vi "Read Message.vi"(11 "LogMessage In":refnum<class "LogMessage.lvclass">) -> (2 "Message":string, 3 "LogMessage Out":refnum<class "LogMessage.lvclass">)   [LabVIEW 2019, in "LogMessage.lvclass"]
uses:
  LogMessage.lvclass
  LogMessage.lvclass/LogMessage.ctl
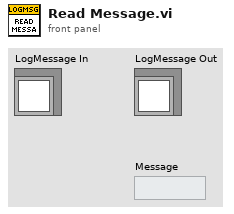
[diagram p1: front panel]
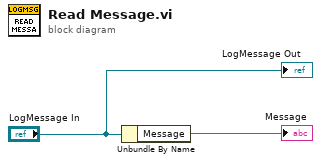
[diagram p0: block diagram]
diagram:
  n1 = Unbundle By Name("LogMessage In") -> ("Message"=→"Message":string)
  "LogMessage Out" <- "LogMessage In"
